vi "GSP_Manager_SCLNServer.vi"() -> ()   [LabVIEW 2015]
uses:
  SystemUtil/Command.ctl
panel:
  in  "Error In":errorcluster={"status"=TRUE, "code"=7, "source"="Open Config Data.vi"}
  out "Message Out":string
  out "Message In":string
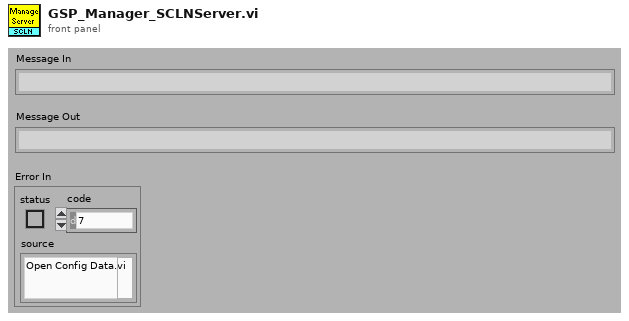
[diagram p1: front panel]
types:
  T1 = typedef "Command.ctl" = cluster{"Command":string, "Parameter":string}
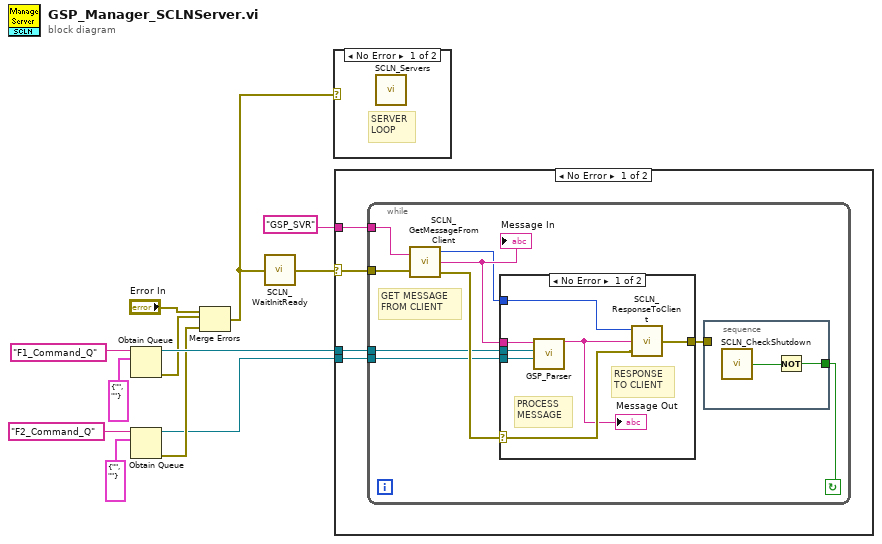
[diagram p0: block diagram]
diagram:
  n1 = Obtain Queue(name (unnamed)="F1_Command_Q", element data type=T1 {"Command"="", "Parameter"=""} ("Command")) -> (queue out=w8:refnum<queue>, error out=w7:errorcluster)  [unwired: 3 in, 1 out]
  n2 = Obtain Queue(name (unnamed)="F2_Command_Q", element data type=T1 {"Command"="", "Parameter"=""} ("Command")) -> (queue out=w1:refnum<queue>, error out=w2:errorcluster)  [unwired: 3 in, 1 out]
  n3 = Merge Errors("Error In", w7, w2) -> (w5:errorcluster)
  n4 = call "SCLN_WaitInitReady.vi"("error in (no error)"=w5) -> ("error out"=w12:errorcluster)
  n5 = case shown="No Error" w5 {
    frame No Error {
      # "SERVER\nLOOP"
      n6 = call "SCLN_Servers.vi"() -> ()  [unwired: 1 out]
    }
    frame Error {
    }
  }
  n7 = case shown="No Error" w12 {
    selector: w12 -> [w15 _]
    tunnel: "GSP_SVR" ("String") -> [w16 _]
    tunnel: w8 -> [w14 _]
    tunnel: w1 -> [w13 _]
    frame No Error {
      n8 = while {
        tunnel: w15 -> [w25]
        tunnel: w16 -> [w20]
        tunnel: w14 -> [w18]
        tunnel: w13 -> [w17]
        stop <- w21 continue-if-true
        # "GET MESSAGE\nFROM CLIENT"
        n9 = call "SCLN_GetMessageFromClient.vi"("Server Name"=w20, "error in (no error)"=w25) -> ("Index for Response"=w23:i32, "Message"=w24:string, "error out"=w19:errorcluster)
        "Message In" <- w24
        n10 = case shown="No Error" w19 {
          selector: w19 -> [w32 w35]
          tunnel: w24 -> [w30 _]
          tunnel: w23 -> [w34 _]
          tunnel: [w33 w35] -> w22
          tunnel: w18 -> [w29 _]
          tunnel: w17 -> [w28 _]
          frame No Error {
            # "PROCESS\nMESSAGE"
            # "RESPONSE\nTO CLIENT"
            n11 = call "GSP_Parser.vi"("Queue F2"=w28, "Queue F1"=w29, "Command"=w30) -> ("Reply"=w31:string)  [unwired: 4 in]
            "Message Out" <- w31
            n12 = call "SCLN_ResponseToClient.vi"("error in (no error)"=w32, "Message"=w31, "Index for Response"=w34) -> ("error out"=w33:errorcluster)
          }
          frame Error {
          }
        }
        n13 = stacked-sequence {
          tunnel: [w26] -> w21
          tunnel: w22 -> [_]
          frame #0 {
            n14 = call "SCLN_CheckShutdown.vi"() -> ("Shutdown"=w27:bool)
            n15 = Not(x=w27) -> (.not. x?=w26:bool)
          }
        }
      }
    }
    frame Error {
    }
  }
